vi "Destroy.vi"(8 "error in (no error)":errorcluster, 11 "Galaxy in":refnum<class "Galaxy.lvclass">) -> (0 "error out":errorcluster)   [LabVIEW 2021, in "Galaxy.lvclass"]
uses:
  Galaxy.lvclass
  Galaxy.lvclass/Galaxy.ctl
  Resource Manager/Resource Manager.lvclass
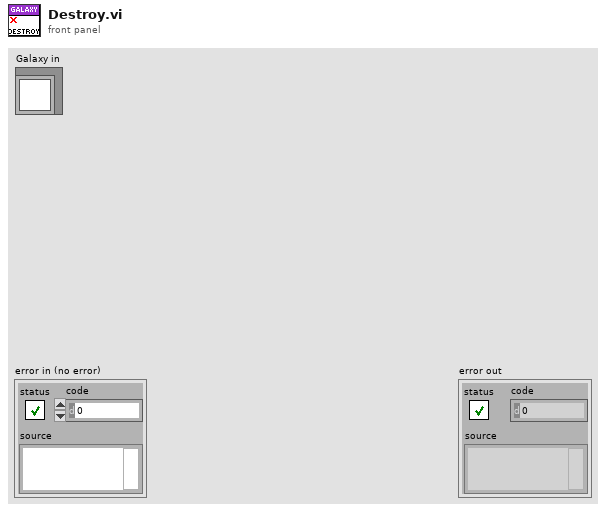
[diagram p1: front panel]
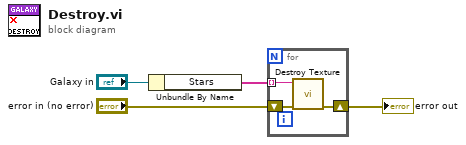
[diagram p0: block diagram]
diagram:
  n1 = Unbundle By Name("Galaxy in") -> ("Stars"=w4:string[])
  n2 = for {
    shift-right: [w6] -> w2
    shift-left: "error in (no error)" -> [w7]
    tunnel: w4 -> [w5] mode=indexing
    n3 = call "Destroy Texture.vi"("error in (no error)"=w7, "Texture Name"=w5) -> ("error out"=w6:errorcluster)  [unwired: 9 in]
  }
  "error out" <- w2
